vi "Sequence.CreateSteps.vi"(4 "Skip":T1, 6 "Step":T3, 8 "error in (no error)":errorcluster, 9 "StepInfo":T1, 10 "Iteration":i32, 11 "Refs":T2) -> (0 "error out":errorcluster, 3 "Refs out":T2)   [LabVIEW 2013, in "Simple Sequence Tools - Editor.lvlib"]
uses:
  Simple Sequence Tools - Editor.lvlib
  Types/Sequence.MainSeqRefs.ctl
  NationalInstruments.VeriStand.RealTimeSequenceDefinitionApi
  Types/Compiled.StepProperties.ctl
  Types/Compiled.IOStateProperties.ctl
  Types/Compiled.StepElementProperties.ctl
  Shared/Types/Channel.Properties.ctl
  Shared/Types/Step.Types.ctl
  Types/Compiled.StepCondition.ctl
  Types/Conditions.OperationTypes.ctl
  Shared/SubVIs/Main.Constants.vi
  Shared/Simple Sequence Tools - Shared.lvlib
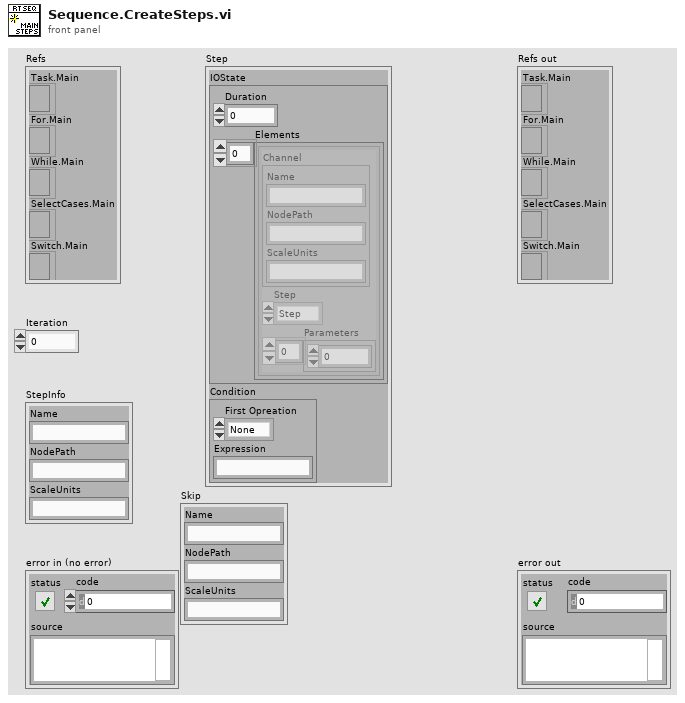
[diagram p1: front panel]
types:
  T1 = typedef "Simple Sequence Tools - Shared.lvlib/Channel.Properties.ctl" = cluster{"Name":string, "NodePath":string, "ScaleUnits":string}
  T2 = typedef "Simple Sequence Tools - Editor.lvlib/Sequence.MainSeqRefs.ctl" = cluster{"Task.Main":refnum<k24>, "For.Main":refnum<k24>, "While.Main":refnum<k24>, "SelectCases.Main":refnum<k24>, "Switch.Main":refnum<k24>}
  T3 = typedef "Simple Sequence Tools - Editor.lvlib/Compiled.StepProperties.ctl" = cluster{"IOState":T4, "Condition":T7}
  T4 = typedef "Simple Sequence Tools - Editor.lvlib/Compiled.IOStateProperties.ctl" = cluster{"Duration":dbl, "Elements":T5[]}
  T5 = typedef "Simple Sequence Tools - Editor.lvlib/Compiled.StepElementProperties.ctl" = cluster{"Channel":T1, "Step":T6, "Parameters":dbl[]}
  T6 = typedef "Simple Sequence Tools - Shared.lvlib/Step.Types.ctl" = enum8{"Step", "iStep", "Ramp", "Unchanged", "Unknown", "Sine"}
  T7 = typedef "Simple Sequence Tools - Editor.lvlib/Compiled.StepCondition.ctl" = cluster{"First Opreation":T8, "Expression":string}
  T8 = typedef "Simple Sequence Tools - Editor.lvlib/Conditions.OperationTypes.ctl" = enum8{"None", "&&", "||"}
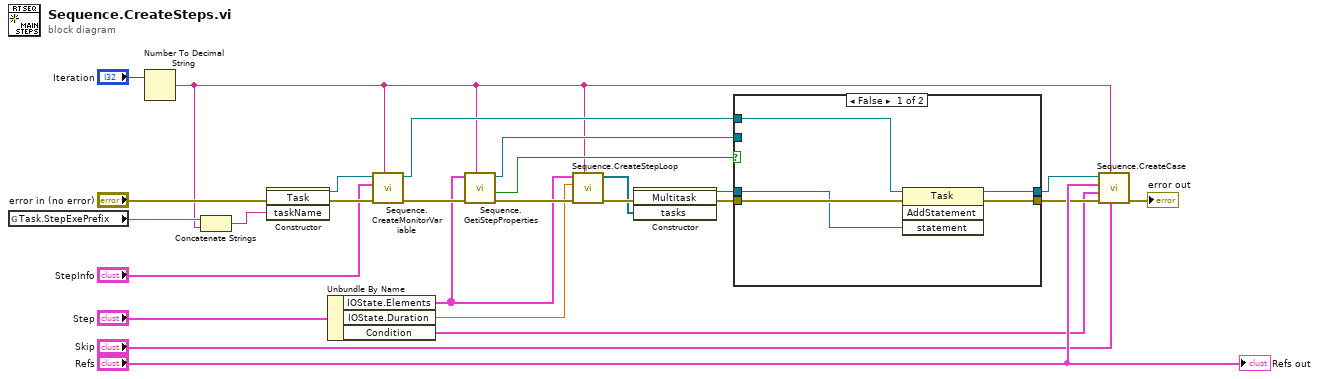
[diagram p0: block diagram]
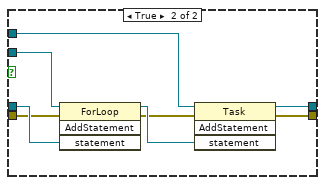
[diagram p2: hidden frame]
diagram:
  n1 = global read "Main.Constants.vi" "Task.StepExePrefix"() -> (w26:string)
  n2 = Number To Decimal String(number="Iteration") -> (decimal integer string=w3:string)  [unwired: 1 in]
  n3 = Concatenate Strings(w26, w3) -> (w17:string)
  n4 = constructor class="Task"(error in="error in (no error)", "taskName"=w17) -> (reference out=w22:refnum<k24>, error out=w21:errorcluster)  [unwired: 2 in, 2 out]
  n5 = Unbundle By Name("Step") -> ("IOState.Elements"=w6:T5[], "IOState.Duration"=w5:dbl, "Condition"=w2:T7)
  n6 = call "Sequence.CreateMonitorVariable.vi"("Iteration"=w3, "error in (no error)"=w21, "StepInfo"="StepInfo", "Task Ref"=w22) -> ("error out"=w23:errorcluster, "Task Ref out"=w24:refnum<k24>)  [unwired: 6 in]
  n7 = call "Sequence.GetiStepProperties.vi"("Iteration"=w3, "error in (no error)"=w23, "Elements"=w6) -> ("error out"=w11:errorcluster, "Step Conatins iStep?"=w14:bool, "iStepForLoop Ref"=w4:refnum<k24>)  [unwired: 6 in]
  n8 = call "Sequence.CreateStepLoop.vi"("Iteration"=w3, "error in (no error)"=w11, "Duration"=w5, "Elements"=w6) -> ("error out"=w10:errorcluster, "Tasks"=w9:refnum<k24>[])  [unwired: 6 in]
  n9 = constructor class="Multitask"(error in=w10, "tasks"=w9) -> (reference out=w12:refnum<k24>, error out=w13:errorcluster)  [unwired: 2 in, 2 out]
  n10 = case shown="False" w14 {
    tunnel: w4 -> [_ w39]
    tunnel: w12 -> [w27 w38]
    tunnel: w13 -> [w30 w37]
    tunnel: [w29 w33] -> w15
    tunnel: [w28 w32] -> w16
    tunnel: w24 -> [w31 w36]
    frame False {
      n11 = invoke class="Task" method="AddStatement"(reference=w31, error in=w30, "statement"=w27) -> (reference out=w28:refnum<k24>, error out=w29:errorcluster)  [unwired: 1 in, 2 out]
    }
    frame True {
      n12 = invoke class="ForLoop" method="AddStatement"(reference=w39, error in=w37, "statement"=w38) -> (reference out=w35:refnum<k24>, error out=w34:errorcluster)  [unwired: 1 in, 2 out]
      n13 = invoke class="Task" method="AddStatement"(reference=w36, error in=w34, "statement"=w35) -> (reference out=w32:refnum<k24>, error out=w33:errorcluster)  [unwired: 1 in, 2 out]
    }
  }
  n14 = call "Sequence.CreateCase.vi"("Skip"="Skip", "Iteration"=w3, "error in (no error)"=w15, "Condition"=w2, "Refs"="Refs", "TaskRef"=w16) -> ("error out"=→"error out":errorcluster)  [unwired: 5 in]
  "Refs out" <- "Refs"
